vi "Functional Test.vi"() -> ()   [LabVIEW 2024]
uses:
  Log Record.ctl
  Logger/Internal Log Levels.ctl
  3ae5ef6d-8e83-4c37-89d5-c4af1027e008.vi
  d7f581ef-27d1-4084-8bbe-9e7418d10964.vi
  d7f581ef-27d1-4084-8bbe-9e7418d10964.vi/a153a250-4fb8-4a99-bb5b-6ccb57f1f631.vi
  d7f581ef-27d1-4084-8bbe-9e7418d10964.vi/a153a250-4fb8-4a99-bb5b-6ccb57f1f631.vi/28727e37-b0d9-407c-a479-ab0b7779cd69.vi
  Formatters/Format String/Format String.lvclass
  C:/Users/Colin/Documents/LabVIEW/Logging/Formatters/Formatter/Formatter.lvclass
  Handlers/String Handler/String Handler.lvclass
  C:/Users/Colin/Documents/LabVIEW/Logging/Handlers/Handler/Handler.lvclass
  Registry/Log.vi
  Logger/Logger.lvclass
  Registry/Registry.lvlib
  Logging.lvlib
panel:
  out "error out":errorcluster
  out "failures":T3(array[cluster]) {"Log Record"."timestamp" format="%<%x %.3X>T"}
  in  "multi-line w/auto-scroll":string
  in  "single line":string
  in  "multi-line":string
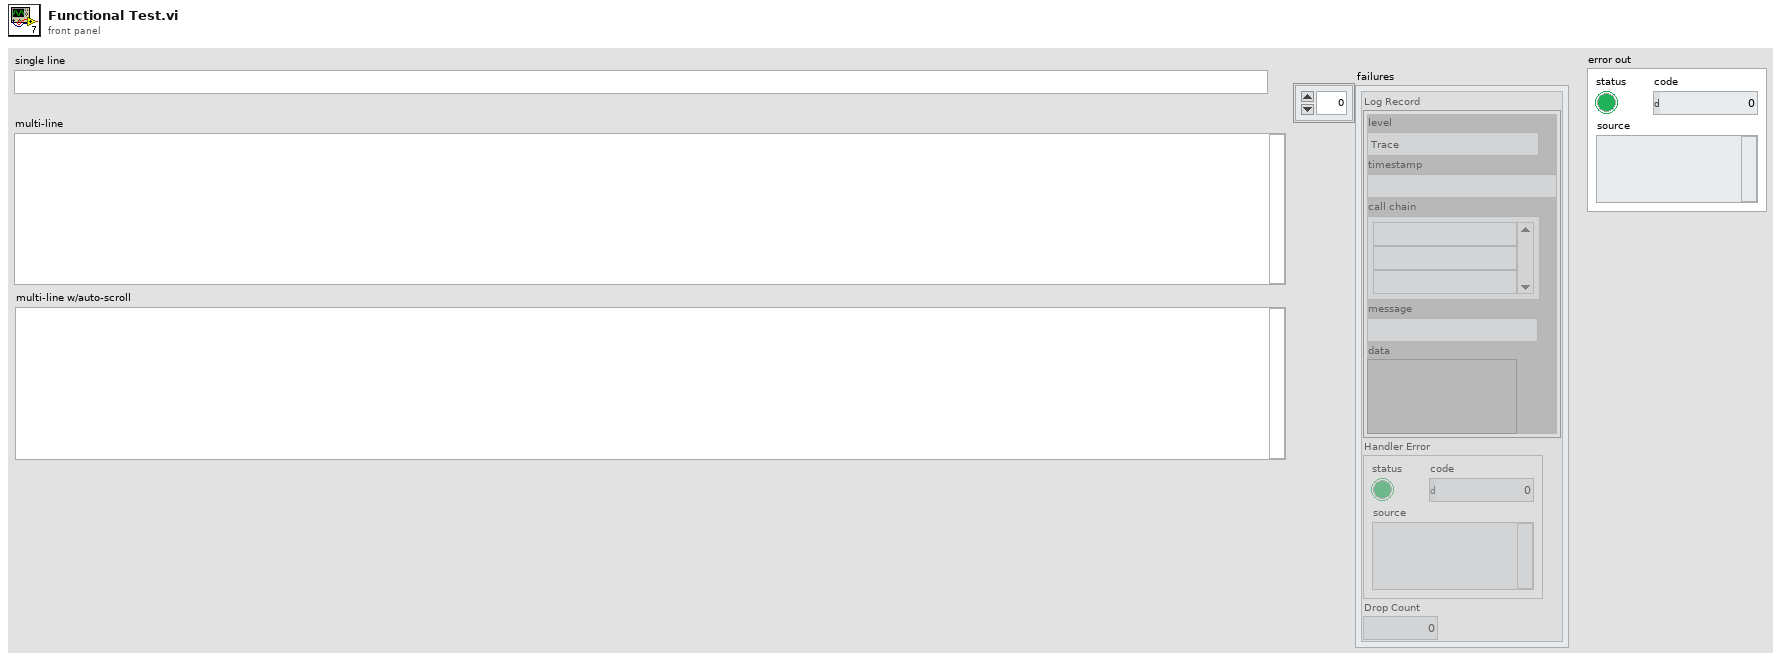
[diagram p1: front panel]
types:
  T1 = typedef "Logging.lvlib/Log Record.ctl" = cluster{"level":T2, "timestamp":timestamp, "call chain":string[], "message":string, "data":variant}
  T2 = typedef "Logging.lvlib/Internal Log Levels.ctl" = enum16{"Trace", "Debug", "Info", "Warning", "Error", "Critical", "Internal"}
  T3 = cluster{"Log Record":T1, "Handler Error":errorcluster, "Drop Count":u32}[]
  T4 = cluster{"Log Record":T1, "Handler Error":errorcluster, "Drop Count":u32}
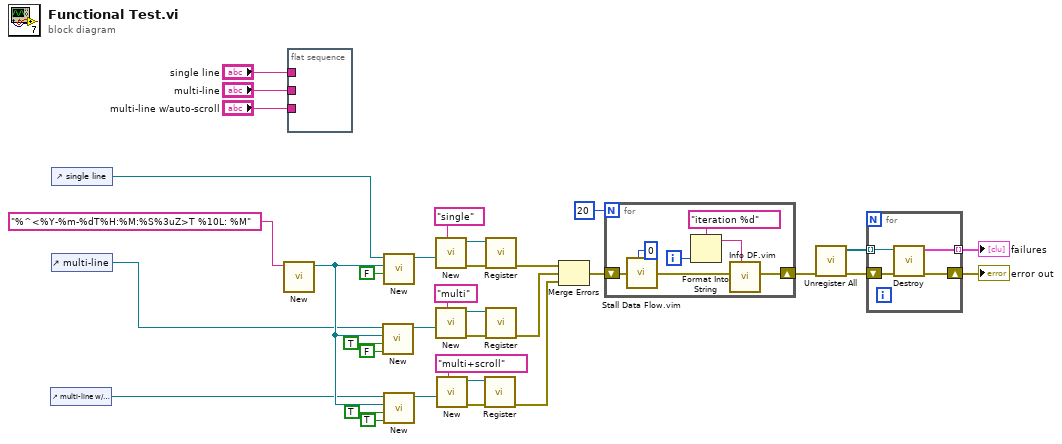
[diagram p0: block diagram]
diagram:
  n1 = control-ref of="multi-line w/auto-scroll"() -> (w27:refnum<vi>)
  n2 = control-ref of="single line"() -> (w29:refnum<vi>)
  n3 = control-ref of="multi-line"() -> (w28:refnum<vi>)
  n4 = call "New.vi"("format string"="%^<%Y-%m-%dT%H:%M:%S%3uZ>T %10L: %M") -> ("new f-string formatter"=w30:refnum<class "Format String.lvclass">)  [unwired: 10 in]
  n5 = flat-sequence {
    tunnel: "single line" -> [_]
    tunnel: "multi-line" -> [_]
    tunnel: "multi-line w/auto-scroll" -> [_]
    frame #0 {
    }
  }
  n6 = call "New.vi"("auto-scroll? (T)"=FALSE, "multi-line? (T)"=TRUE, "formatter (format string)"=w30, "string control"=w28) -> ("new string handler"=w24:refnum<class "String Handler.lvclass">)  [unwired: 7 in]
  n7 = call "New.vi"("multi-line? (T)"=FALSE, "formatter (format string)"=w30, "string control"=w29) -> ("new string handler"=w26:refnum<class "String Handler.lvclass">)  [unwired: 8 in]
  n8 = call "New.vi"("auto-scroll? (T)"=TRUE, "multi-line? (T)"=TRUE, "formatter (format string)"=w30, "string control"=w27) -> ("new string handler"=w21:refnum<class "String Handler.lvclass">)  [unwired: 7 in]
  n9 = call "New.vi"("name (\"Default\")"="single" ("name (\"Default\")"), "log handler (file handler)"=w26) -> ("error out"=w19:errorcluster, "logger"=w20:refnum<class "Logger.lvclass">)  [unwired: 8 in]
  n10 = call "New.vi"("name (\"Default\")"="multi" ("name (\"Default\")"), "log handler (file handler)"=w24) -> ("error out"=w17:errorcluster, "logger"=w18:refnum<class "Logger.lvclass">)  [unwired: 8 in]
  n11 = call "New.vi"("name (\"Default\")"="multi+scroll" ("name (\"Default\")"), "log handler (file handler)"=w21) -> ("error out"=w15:errorcluster, "logger"=w16:refnum<class "Logger.lvclass">)  [unwired: 8 in]
  n12 = call "Register.vi"("error in (no error)"=w15, "logger in"=w16) -> ("error out"=w12:errorcluster)  [unwired: 9 in]
  n13 = call "Register.vi"("error in (no error)"=w19, "logger in"=w20) -> ("error out"=w14:errorcluster)  [unwired: 9 in]
  n14 = call "Register.vi"("error in (no error)"=w17, "logger in"=w18) -> ("error out"=w13:errorcluster)  [unwired: 9 in]
  n15 = Merge Errors(w14, w13, w12) -> (w11:errorcluster)
  n16 = for {
    N: 20 -> [_]
    shift-right: [w36] -> w9
    shift-left: w11 -> [w41]
    i -> [w39]
    n17 = call "Stall Data Flow.vim"("value in"=w41, "milliseconds to wait"=u32 0) -> ("value out"=w40:errorcluster)  [unwired: 1 out]
    n18 = Format Into String(format string="iteration %d", w39) -> (resulting string=w37:string)  [unwired: 2 in, 1 out]
    n19 = call "Info DF.vim"("message"=w37, "dataflow in"=w40) -> ("dataflow out"=w36:errorcluster)  [unwired: 9 in]
  }
  n20 = call "Unregister All.vi"("error in (no error)"=w9) -> ("error out"=w8:errorcluster, "loggers"=w7:refnum<class "Logger.lvclass">[])  [unwired: 9 in]
  n21 = for {
    tunnel: w7 -> [w45] mode=indexing
    tunnel: [w44] -> w6 mode=indexing
    shift-right: [w43] -> w5
    shift-left: w8 -> [w46]
    n22 = call "Destroy.vi"("error in (no error)"=w46, "logger in"=w45) -> ("error out"=w43:errorcluster, "fail info"=w44:T4)  [unwired: 8 in]
  }
  "failures" <- w6
  "error out" <- w5
